vi "CMDCore循环启用.vi"(0 "MainPage输入":refnum<class "MainPage.lvclass">) -> (14 "MainPage输出":refnum<class "MainPage.lvclass">)   [LabVIEW 2019, in "MainPage.lvlib" / "MainPage.lvclass"]
uses:
  MainPage.lvclass
  D:/Program Files (x86)/National Instruments/LabVIEW 2019/vi.lib/ActorFramework/Actor/Actor.lvclass
  <vilib>/ActorFramework/Actor/Actor.lvclass/Actor.ctl
  <vilib>/ActorFramework/Message Enqueuer/Message Enqueuer.lvclass/Message Enqueuer.ctl
  MainPage.lvclass/MainPage.ctl
  <vilib>/ActorFramework/Message Enqueuer/Init from Existing Queue.vi
  D:/Program Files (x86)/National Instruments/LabVIEW 2019/vi.lib/ActorFramework/Message/Message.lvclass
  <vilib>/ActorFramework/Message Enqueuer/Message Enqueuer.lvclass
  <vilib>/ActorFramework/Actor/Actor.lvclass
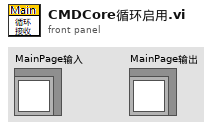
[diagram p1: front panel]
types:
  T1 = typedef "MainPage.lvlib/MainPage.lvclass/通用配置选项.ctl" = cluster{"ModBusRTU反馈":enum32{"模拟反馈", "无反馈", "错误反馈"}, "侦听周期":u32, "跳转反馈":bool, "报文记录数量":u16, "客服端新增模式":enum32{"单端模式", "多端共存"}}
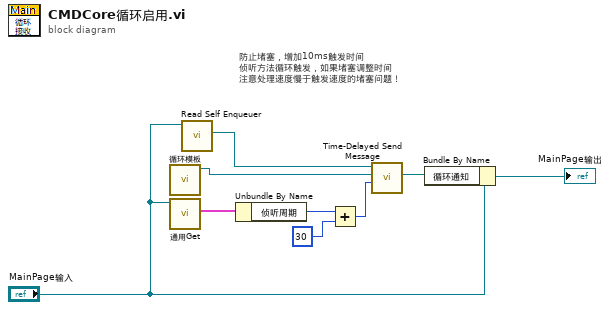
[diagram p0: block diagram]
diagram:
  # "防止堵塞，增加10ms触发时间\n侦听方法循环触发，如果堵塞调整时间\n注意处理速度慢于触发速度的堵塞问题！"
  n1 = call "循环模板.vi"() -> ("CMDCore消息 输出"=w2:refnum<class "CMDCore消息.lvclass">)  [unwired: 10 in, 1 out]
  n2 = call-dynamic "通用Get.vi"("MainPage 输入"="MainPage输入") -> ("通用配置"=w7:T1)  [unwired: 6 in, 4 out]
  n3 = call <vilib>:"Read Self Enqueuer.vi"("Actor"="MainPage输入") -> ("Self Enqueuer"=w3:refnum<class "Message Enqueuer.lvclass">)  [unwired: 10 in]
  n4 = Unbundle By Name(w7) -> ("侦听周期"=w4:u32)
  n5 = Add(x=w4, y=u32 30) -> (x+y=w6:u32)
  n6 = call <vilib>:"Time-Delayed Send Message.vi"("Milliseconds To Wait"=w6, "Message"=w2, "Message Enqueuer"=w3) -> ("Delivery Notifier"=w1:refnum<notifier>)  [unwired: 7 in, 1 out]
  n7 = Bundle By Name(cluster="MainPage输入", "循环通知"=w1) -> (→"MainPage输出":refnum<class "MainPage.lvclass">)
